vi "main_ctrl.vi"(8 "error in":errorcluster) -> (0 "error out":errorcluster caption="Error")   [LabVIEW 2013]
uses:
  <vilib>/Rock Robotics/WPI/DriverStation/WPI_DriverStationRobotMode2.ctl
  typedefs/fg_typedef.ctl
  typedefs/vision enable.ctl
  typedefs/subStates.ctl
  typedefs/singleUseSubstate.ctl
  <vilib>/Rock Robotics/WPI/Solenoid/WPI_SolenoidValue.ctl
  <vilib>/Rock Robotics/WPI/Compressor/WPI_CompressorGetSetRefNum.vi
  <vilib>/Rock Robotics/WPI/RobotDrive/WPI_RobotDriveGetSetRefNum.vi
  <vilib>/Rock Robotics/WPI/RobotDrive/WPI_RobotDriveArcadeDrive_Standard(NoSaturation).vi
  <vilib>/Rock Robotics/WPI/Solenoid/WPI_SolenoidSetEnum.vi
  typedefs/vision data.ctl
panel:
  out "Robot Mode":T1
  out "Vision SPI":u32
  out "Vision IPS":dbl
  out "Main IPS":dbl
  out "Main SPI":u32
  # "MAIN CONTROL"
  # "holds robot control code - dual parallel state machine"
  # "SPI: milliseconds per iteration\nIPS: iterations per second"
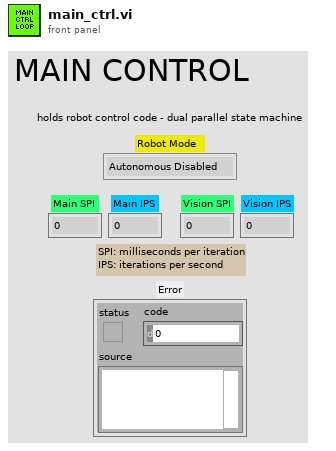
[diagram p1: front panel]
types:
  T1 = typedef "WPI_DriverStationRobotMode2.ctl" = enum16{"Autonomous Disabled", "Autonomous Enabled", "Teleop Disabled", "Teleop Enabled", "Timeout", "Finish", "Test Disabled", "Test Enabled"}
  T2 = typedef "fg_typedef.ctl" = enum16{"Get", "Set"}
  T3 = typedef "WPI_DigitalInputDevRef.ctl" = cluster{"DevStatus":errorcluster, "DIO Channel":T4, "Digital Module":T5}
  T4 = typedef "FPGA_DIOChannel.ctl" = enum8{"DIO 1", "DIO 2", "DIO 3", "DIO 4", "DIO 5", "DIO 6", "DIO 7", "DIO 8", "DIO 9", "DIO 10", "DIO 11", "DIO 12", "DIO 13", "DIO 14", "Invalid"}
  T5 = typedef "FPGA_TypedefDigitalModule.ctl" = enum16{"Digital Module 1", "Digital Module 2"}
  T6 = typedef "WPI_RobotDriveDevRef.ctl" = cluster{"DevStatus":errorcluster, "Motors[]":T7[], "Square Inputs":bool, "Max Output":dbl, "Isochronous":bool}
  T7 = typedef "WPI_MotorControlDeviceRef.ctl" = cluster{"DeviceStatus":errorcluster, "Type":enum16{"PWM", "CAN"}, "PWM":cluster{"Digital Module":T5, "PWM Channel":T8, "DeadBand":T9}, "CAN":cluster{"Device Number":u8, "Control Mode":T10, "Semaphore":T11, "Max Vout":dbl}, "Invert":bool, "TransformRef":T12, "InvTransformRef":T12}
  T8 = typedef "FPGA_DIOPWMChannel.ctl" = enum8{"PWM 1", "PWM 2", "PWM 3", "PWM 4", "PWM 5", "PWM 6", "PWM 7", "PWM 8", "PWM 9", "PWM 10", "Invalid"}
  T9 = typedef "WPI_PWMDeadband.ctl" = cluster{"Name":string, "maxPositivePwm":i32, "minPositivePwm":i32, "centerPwm":i32, "maxNegativePwm":i32, "minNegativePwm":i32, "angularRange":u16}
  T10 = typedef "WPI_CANJaguar_ControlMode.ctl" = enum8{"Percent VBus", "Current", "Speed", "Position", "Voltage"}
  T11 = typedef "Semaphore RefNum" = refnum<k1>
  T12 = typedef "WPI_PWMTransform_ConPane.ctl" = refnum<vi>
  T13 = typedef "WPI_SolenoidDevRef.ctl" = cluster{"DevStatus":errorcluster, "Solenoid Module":T14, "Forward Solenoid Channel":T15, "Reverse Solenoid Channel":T15}
  T14 = typedef "FPGA_TypedefSolenoidModule.ctl" = enum16{"Solenoid Module 1", "Solenoid Module 2"}
  T15 = typedef "WPI_SolenoidChannel.ctl" = enum8{"Solenoid 1", "Solenoid 2", "Solenoid 3", "Solenoid 4", "Solenoid 5", "Solenoid 6", "Solenoid 7", "Solenoid 8", "Invalid"}
  T16 = typedef "WPI_EncoderDevRef.ctl" = cluster{"DevStatus":errorcluster, "EncoderIndex":T17, "CounterIndex":T18, "DistancePerCount":dbl, "Decoding Type":T19}
  T17 = typedef "FPGA_EncoderIdx.ctl" = enum8{"Enc 0", "Enc 1", "Enc 2", "Enc 3", "Invalid"}
  T18 = typedef "FPGA_CounterCtrSystemIndex.ctl" = enum8{"Ctr 0", "Ctr 1", "Ctr 2", "Ctr 3", "Ctr 4", "Ctr 5", "Ctr 6", "Ctr 7", "Invalid"}
  T19 = typedef "WPI_EncoderType.ctl" = enum16{"1x", "2x", "4x"}
  T20 = typedef "vision data.ctl" = cluster{"x":dbl, "y":dbl, "area":dbl, "width":dbl, "height":dbl, "Hot Goal Present?":bool, "distance":dbl}
  T21 = typedef "vision enable.ctl" = enum16{"Enable", "Disable", "Stop"}
  T22 = typedef "WPI_CameraDevRef.ctl" = cluster{"Camera Address":string, "CameraStatus":errorcluster, "Acquire Image Notifier":refnum<notifier>}
  T23 = typedef "IMAQ Image.ctl" = refnum<image>
  T24 = cluster{"Vision mSPI":u32, "Main mSPI":u32, "Dash mSPI":u32}
  T25 = typedef "WPI_CompressorDevRef.ctl" = cluster{"DevStatus":errorcluster, "DigitalInputDevRef":T3, "RelayDevRef":T26}
  T26 = typedef "WPI_RelayDevRef.ctl" = cluster{"DevStatus":errorcluster, "Relay Channel":T27, "Digital Module":T5, "Relay Direction":T28}
  T27 = typedef "FPGA_DIORelayChannel.ctl" = enum8{"Relay 1", "Relay 2", "Relay 3", "Relay 4", "Relay 5", "Relay 6", "Relay 7", "Relay 8", "Invalid"}
  T28 = typedef "WPI_RelayDirection.ctl" = enum16{"Both directions", "Forward only", "Reverse only"}
  T29 = typedef "WPI_SolenoidValue.ctl" = enum16{"Off", "On", "Forward", "Reverse"}
  T30 = typedef "singleUseSubstate.ctl" = enum16{"null", "wait", "shift high", "shift low", "extend shooter", "retract shooter", "latch", "unlatch", "end"}
  T31 = typedef "WPI_DriverStationDerivedRobotMode.ctl" = enum16{"Init", "Execute", "Stop"}
  T32 = typedef "subStates.ctl" = enum16{"null", "wait", "driver control", "auto", "manual override", "hold position", "rotate", "pickup", "pass", "load", "goto shoot", "shoot high goal", "shoot low goal", "cancel arm", "cancel shooter", "end"}
  T33 = typedef "Loop 2 Datatype.ctl" = cluster{"State":T32, "Waiting Loop":i32, "State to Wait For":i32, "Loop ID":i32, "Exit Value":i32, "Joystick Y":dbl, "Joystick Z":dbl}
  T34 = typedef "Loop 1 Datatype.ctl" = cluster{"State":T32, "Waiting Loop":i32, "State to Wait For":i32, "Loop ID":i32, "Exit Value":i32}
  T35 = typedef "Loop 3 Datatype.ctl" = cluster{"State":T32, "Waiting Loop":i32, "State to Wait For":i32, "Loop ID":i32, "Exit Value":i32, "Joystick Y":dbl, "Tune Setpoint":cluster{"Increment":bool, "Decrement":bool}}
  T36 = typedef "Loop 0 Datatype.ctl" = cluster{"State":T32, "Waiting Loop":i32, "State to Wait For":i32, "Loop ID":i32, "Exit Value":i32, "X Axis":dbl, "Y Axis":dbl, "Z Axis":dbl}
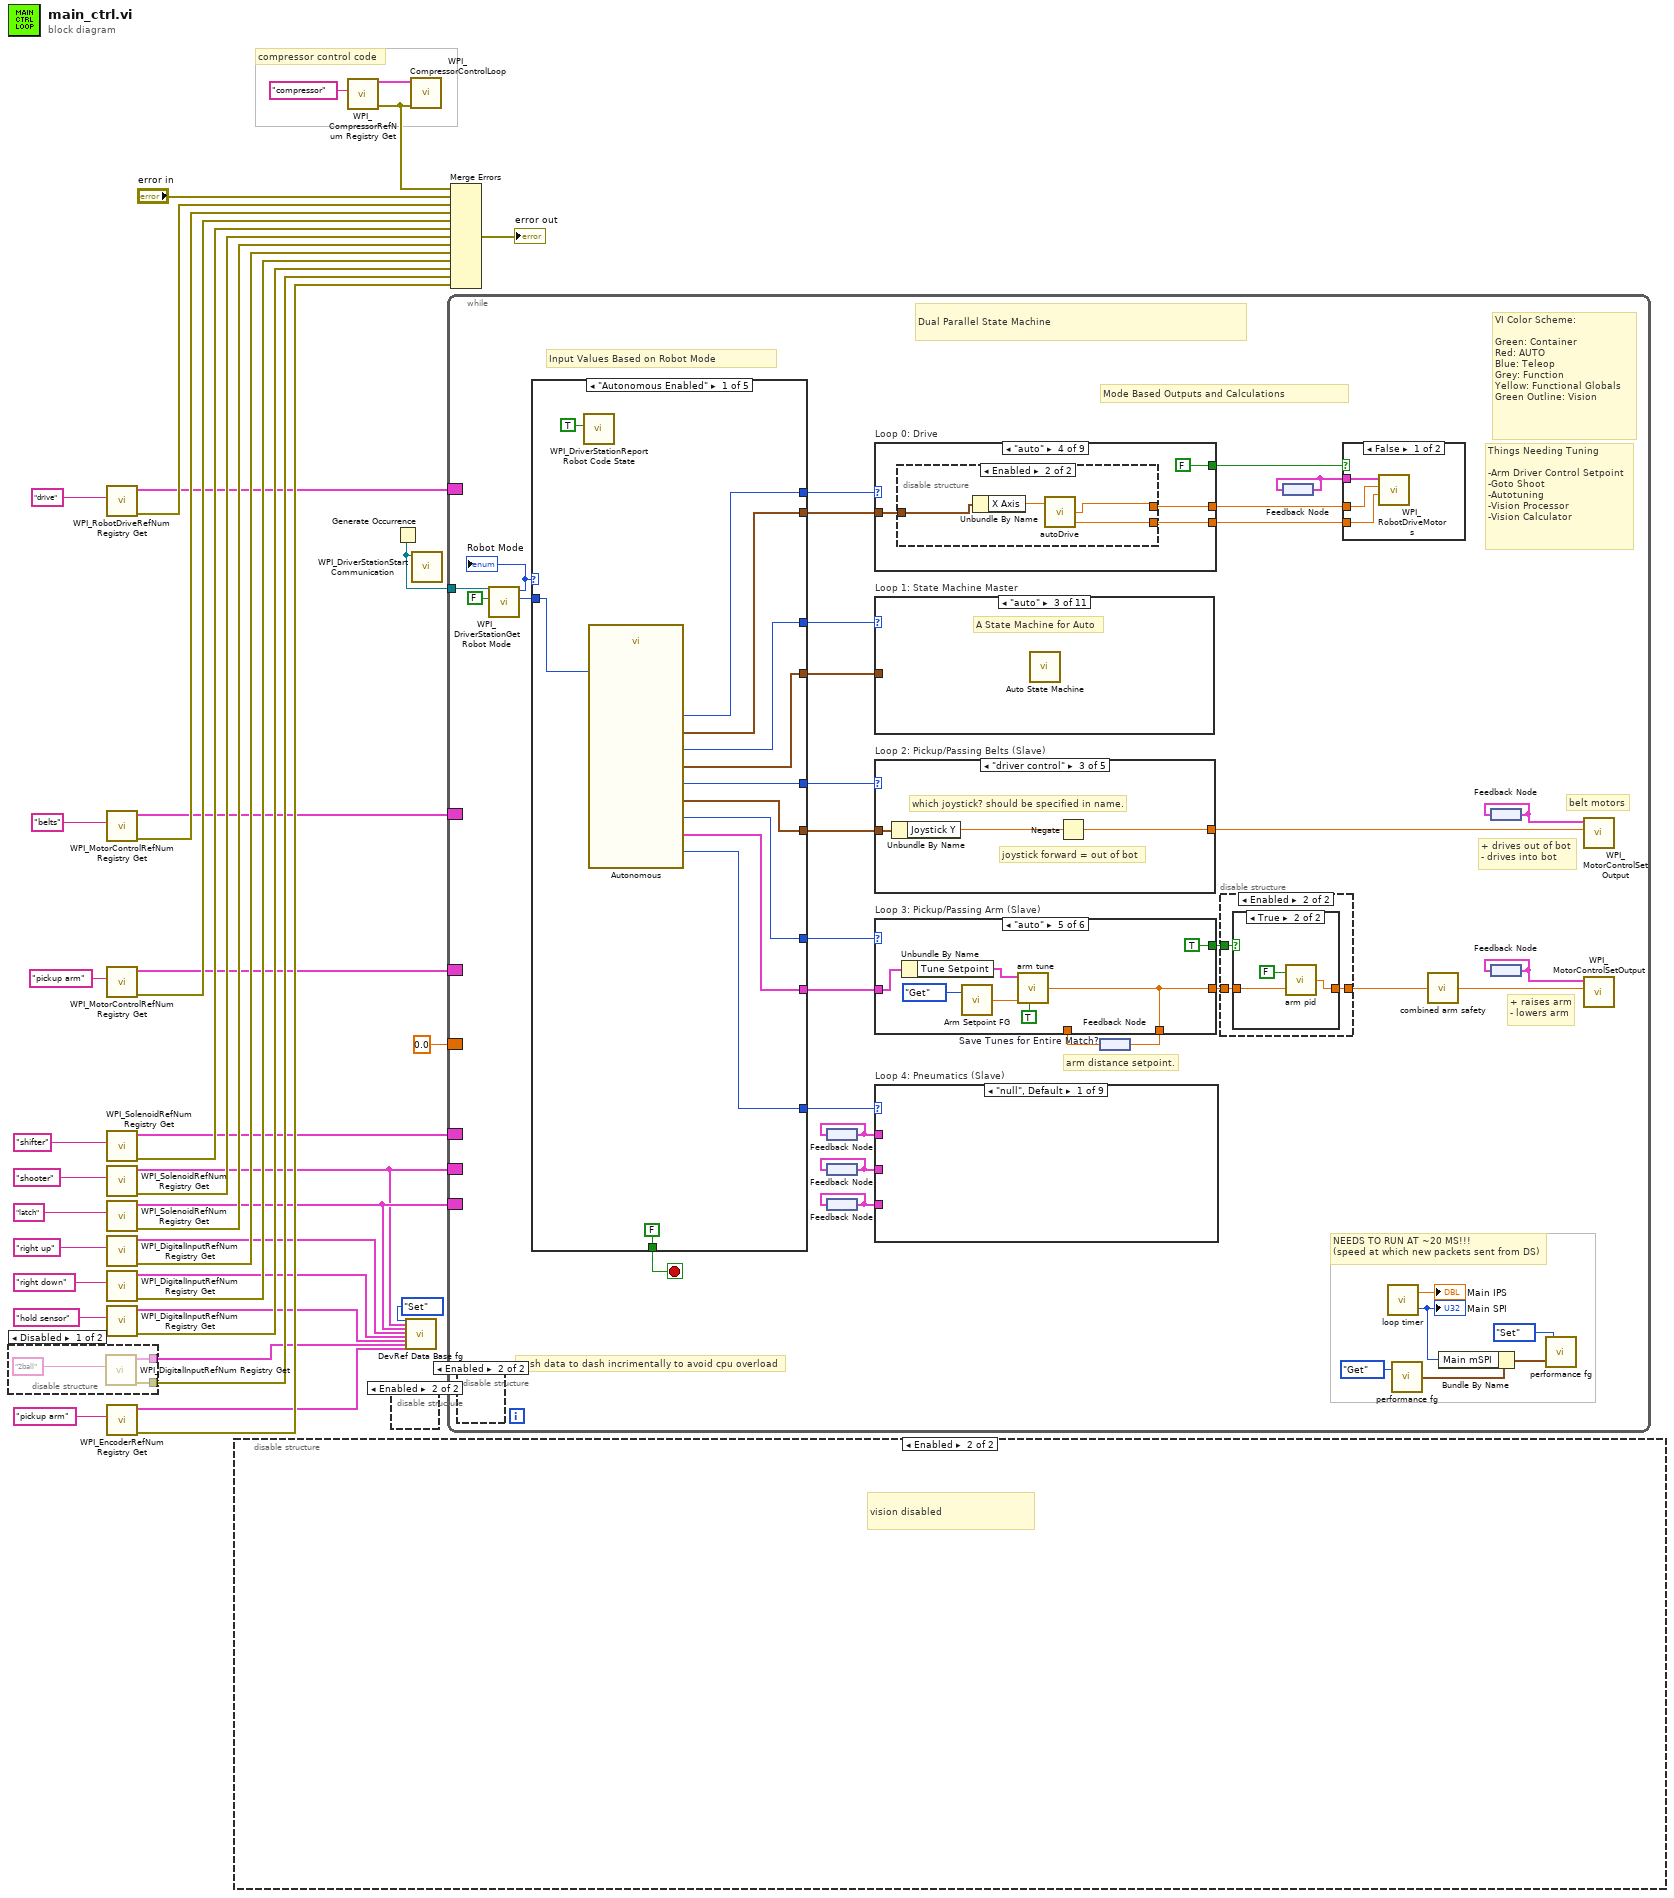
[diagram p0: block diagram]
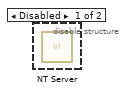
[diagram p3: hidden frame]
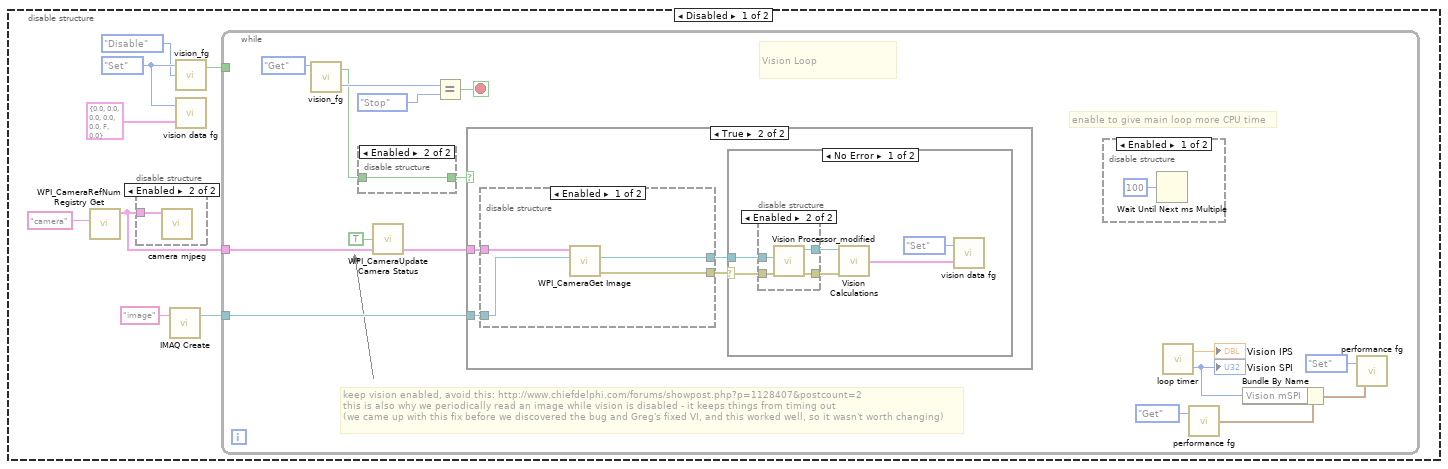
[diagram p4: hidden frame]
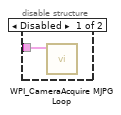
[diagram p5: hidden frame]
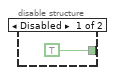
[diagram p6: hidden frame]
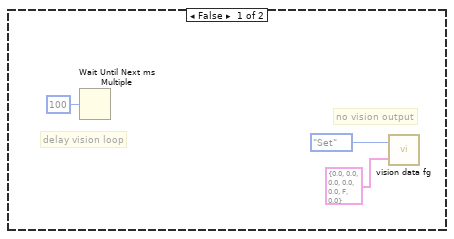
[diagram p8: hidden frame]
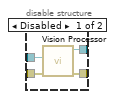
[diagram p9: hidden frame]
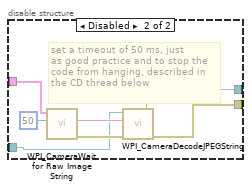
[diagram p11: hidden frame]
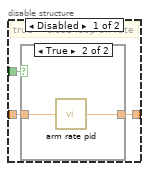
[diagram p12: hidden frame]
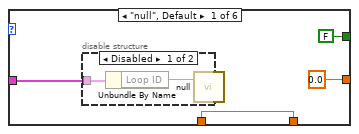
[diagram p15: hidden frame]
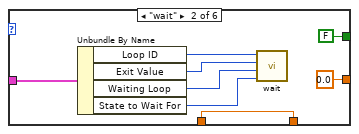
[diagram p17: hidden frame]
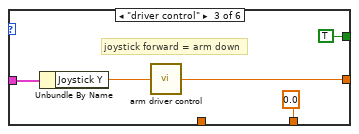
[diagram p18: hidden frame]
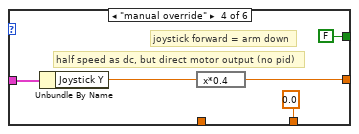
[diagram p19: hidden frame]
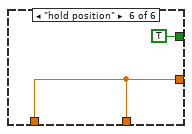
[diagram p20: hidden frame]
diagram:
  # "compressor control code"
  n1 = disable-structure shown="Disabled" {
    disable-tunnel: [w43 _] -> w39
    disable-tunnel: [w41 _] -> w7
    frame Disabled {
      n2 = call <vilib>:"WPI_DigitalInputRefNum Registry Get.vi"("refnum name"="2ball") -> ("error out"=w43:errorcluster, "DigitalInputDevRef"=w41:T3)  [unwired: 9 in]
    }
    frame Enabled {
    }
  }
  n3 = call <vilib>:"WPI_RobotDriveRefNum Registry Get.vi"("refnum name"="drive") -> ("error out"=w38:errorcluster, "RobotDriveDevRef"=w26:T6)  [unwired: 9 in]
  n4 = call <vilib>:"WPI_MotorControlRefNum Registry Get.vi"("refnum name"="belts") -> ("error out"=w37:errorcluster, "MotorControlDevRef"=w5:T7)  [unwired: 9 in]
  n5 = call <vilib>:"WPI_MotorControlRefNum Registry Get.vi"("refnum name"="pickup arm") -> ("error out"=w36:errorcluster, "MotorControlDevRef"=w17:T7)  [unwired: 9 in]
  n6 = call <vilib>:"WPI_SolenoidRefNum Registry Get.vi"("refnum name"="shifter") -> ("error out"=w35:errorcluster, "SolenoidDevRef"=w24:T13)  [unwired: 9 in]
  n7 = call <vilib>:"WPI_SolenoidRefNum Registry Get.vi"("refnum name"="shooter") -> ("error out"=w34:errorcluster, "SolenoidDevRef"=w3:T13)  [unwired: 9 in]
  n8 = call <vilib>:"WPI_SolenoidRefNum Registry Get.vi"("refnum name"="latch") -> ("error out"=w33:errorcluster, "SolenoidDevRef"=w4:T13)  [unwired: 9 in]
  n9 = call <vilib>:"WPI_DigitalInputRefNum Registry Get.vi"("refnum name"="right up") -> ("error out"=w32:errorcluster, "DigitalInputDevRef"=w2:T3)  [unwired: 9 in]
  n10 = call <vilib>:"WPI_DigitalInputRefNum Registry Get.vi"("refnum name"="right down") -> ("error out"=w31:errorcluster, "DigitalInputDevRef"=w1:T3)  [unwired: 9 in]
  n11 = call <vilib>:"WPI_DigitalInputRefNum Registry Get.vi"("refnum name"="hold sensor") -> ("error out"=w30:errorcluster, "DigitalInputDevRef"=w11:T3)  [unwired: 9 in]
  n12 = call <vilib>:"WPI_EncoderRefNum Registry Get.vi"("refnum name"="pickup arm") -> ("error out"=w40:errorcluster, "EncoderDevRef"=w6:T16)  [unwired: 9 in]
  n13 = disable-structure shown="Enabled" {
    frame Disabled {
      w49 = fg_typedef."Set" ("Enum")
      n14 = call <vilib>:"WPI_CameraRefNum Registry Get.vi"("refnum name"="camera") -> ("CameraDevRef"=w46:T22)  [unwired: 9 in, 1 out]
      n15 = disable-structure shown="Enabled" {
        disable-tunnel: w46 -> [w52 w53]
        frame Disabled {
          n16 = call <vilib>:"WPI_CameraAcquire MJPG Loop.vi"("CameraDevRef"=w52) -> ()  [unwired: 11 in]
        }
        frame Enabled {
          n17 = call "camera mjpeg.vi"("CameraDevRef"=w53) -> ()  [unwired: 11 in]
        }
      }
      n18 = call "IMAQ Create"("Image Name"="image") -> ("New Image"=w51:T23)  [unwired: 4 in, 1 out]
      n19 = call "vision_fg.vi"("Action"=vision_enable."Disable", "Menu"=w49) -> ("Enabled?"=w50:bool)  [unwired: 1 in, 1 out]
      n20 = call "vision data fg.vi"("Input"=T20 {"x"=0.0, "y"=0.0, "area"=0.0, "width"=0.0, "height"=0.0, "Hot Goal Present?"=FALSE, "distance"=0.0} ("Cluster"), "Menu"=w49) -> ()  [unwired: 1 out]
      n21 = while {
        tunnel: w51 -> [w68]
        tunnel: w46 -> [w67]
        tunnel: w50 -> [_]
        stop <- w69 stop-if-true
        # "keep vision enabled, avoid this: http://www.chiefdelphi.com/forums/showpost.php?p=1128407&postcount=2\nthis is also why we periodically read an image while vision is disabled - it keeps things from timing out\n(we came up with this fix before we discovered the bug and Greg's fixed VI, and this worked well, so it wasn't worth changing)"
        # "enable to give main loop more CPU time"
        # "Vision Loop"
        n22 = call "vision_fg.vi"("Menu"=fg_typedef."Get" ("Enum")) -> ("State Out"=w63:T21, "Enabled?"=w54:bool)  [unwired: 2 in]
        n23 = disable-structure shown="Enabled" {
          disable-tunnel: [TRUE w71] -> w55
          disable-tunnel: w54 -> [_ w71]
          frame Disabled {
          }
          frame Enabled {
          }
        }
        n24 = call <vilib>:"WPI_CameraUpdate Camera Status.vi"("CameraDevRef In"=w67, "Enable Vision"=TRUE) -> ("CameraDevRef Out"=w66:T22)  [unwired: 3 in]
        n25 = Equal?(x=w63, y=vision_enable."Stop") -> (x = y?=w69:bool)
        n26 = case shown="True" w55 {
          tunnel: w68 -> [_ w79]
          tunnel: w66 -> [_ w78]
          frame False {
            # "no vision output"
            # "delay vision loop"
            n27 = Wait Until Next ms Multiple(millisecond multiple=u32 100) -> ()  [unwired: 1 out]
            n28 = call "vision data fg.vi"("Input"=T20 {"x"=0.0, "y"=0.0, "area"=0.0, "width"=0.0, "height"=0.0, "Hot Goal Present?"=FALSE, "distance"=0.0} ("Cluster"), "Menu"=fg_typedef."Set" ("Enum")) -> ()  [unwired: 1 out]
          }
          frame True {
            n29 = disable-structure shown="Enabled" {
              disable-tunnel: w79 -> [w96 w100]
              disable-tunnel: w78 -> [w97 w102]
              disable-tunnel: [w95 w99] -> w77
              disable-tunnel: [w94 w98] -> w76
              frame Enabled {
                n30 = call <vilib>:"WPI_CameraGet Image.vi"("Image"=w96, "CameraDevRef"=w97) -> ("error out"=w94:errorcluster, "Image Out"=w95:T23)  [unwired: 7 in, 1 out]
              }
              frame Disabled {
                # "set a timeout of 50 ms, just\nas good practice and to stop the \ncode from hanging, described in \nthe CD thread below"
                n31 = call <vilib>:"WPI_CameraWait for Raw Image String.vi"("Timeout in ms (-1)"=50, "CameraDevRef"=w102) -> ("error out"=w104:errorcluster, "String"=w103:string)  [unwired: 3 in, 5 out]
                n32 = call <vilib>:"WPI_CameraDecodeJPEGString.vi"("error in"=w104, "Compressed Image"=w103, "Image In"=w100) -> ("error out"=w98:errorcluster, "Image Out"=w99:T23)  [unwired: 3 out]
              }
            }
            n33 = case shown="No Error" w76 {
              selector: w76 -> [w84 _]
              tunnel: w77 -> [w83 _]
              frame No Error {
                n34 = disable-structure shown="Enabled" {
                  disable-tunnel: w84 -> [w89 w92]
                  disable-tunnel: w83 -> [w88 w93]
                  disable-tunnel: [w87 w90] -> w82
                  disable-tunnel: [w86 w91] -> w81
                  frame Disabled {
                    n35 = call "Vision Processor.vi"("error in"=w89, "Image In"=w88) -> ("error out"=w86:errorcluster, "Image Out"=w87:T23)  [unwired: 5 in]
                  }
                  frame Enabled {
                    n36 = call "Vision Processor_modified.vi"("error in"=w92, "Image In"=w93) -> ("error out"=w91:errorcluster, "Image Out"=w90:T23)  [unwired: 5 in]
                  }
                }
                n37 = call "Vision Calculations.vi"("Image In"=w82, "error in"=w81) -> ("Vision Data"=w80:T20)  [unwired: 3 in]
                n38 = call "vision data fg.vi"("Input"=w80, "Menu"=fg_typedef."Set" ("Enum")) -> ()  [unwired: 1 out]
              }
              frame Error {
              }
            }
          }
        }
        n39 = disable-structure shown="Enabled" {
          frame Enabled {
            n40 = Wait Until Next ms Multiple(millisecond multiple=u32 100) -> ()  [unwired: 1 out]
          }
          frame Disabled {
          }
        }
        n41 = call "loop timer.vi"() -> ("IPS"=→"Vision IPS":dbl, "SPI"=w61:u32)  [unwired: 1 in]
        "Vision SPI" <- w61
        n42 = call "performance fg.vi"("Menu"=fg_typedef."Get") -> ("Output"=w59:T24)  [unwired: 1 in]
        n43 = Bundle By Name(cluster=w59, "Vision mSPI"=w61) -> (w58:T24)
        n44 = call "performance fg.vi"("Input"=w58, "Menu"=fg_typedef."Set") -> ()  [unwired: 1 out]
      }
    }
    frame Enabled {
      # "vision disabled"
    }
  }
  n45 = call <vilib>:"WPI_CompressorRefNum Registry Get.vi"("refnum name"="compressor") -> ("error out"=w10:errorcluster, "CompressorDevRef"=w25:T25)  [unwired: 9 in]
  n46 = disable-structure shown="Enabled" {
    frame Disabled {
      n47 = call <vilib>:"NT Server.vi"() -> ()  [unwired: 12 in]
    }
    frame Enabled {
    }
  }
  n48 = Generate Occurrence() -> (w22:refnum<k4>)
  n49 = call "DevRef Data Base fg.vi"("Menu"=fg_typedef."Set", "Shooter Solenoid DevRef"=w3, "Latch Solenoid DevRef"=w4, "Right Up DevRef"=w2, "Right Down DevRef"=w1, "Hold Sensor DevRef"=w11, "2 Ball DevRef"=w7, "Arm Encoder DevRef"=w6) -> ()  [unwired: 17 in, 3 out]
  n50 = call <vilib>:"WPI_CompressorControlLoop.vi"("error in (no error)"=w10, "CompressorDevRef"=w25) -> ()  [unwired: 10 in]
  n51 = call <vilib>:"WPI_DriverStationStart Communication.vi"("occurrence"=w22) -> ()  [unwired: 11 in]
  n52 = while {
    tunnel: w22 -> [w120]
    border: w26 -> [_]
    border: w24 -> [_]
    border: w4 -> [_]
    border: w3 -> [_]
    border: w5 -> [_]
    border: w17 -> [_]
    border: 0.0 ("setpoint") -> [_]
    stop <- w137 stop-if-true
    # "arm distance setpoint."
    # "push data to dash incrimentally to avoid cpu overload"
    # "Things Needing Tuning\n\n-Arm Driver Control Setpoint\n-Goto Shoot\n-Autotuning\n-Vision Processor\n-Vision Calculator"
    # "+ raises arm\n- lowers arm"
    # "+ drives out of bot\n- drives into bot"
    # "belt motors"
    # "VI Color Scheme:\n\nGreen: Container\nRed: AUTO\nBlue: Teleop\nGrey: Function\nYellow: Functional Globals\nGreen Outline: Vision"
    # "Input Values Based on Robot Mode"
    # "Mode Based Outputs and Calculations"
    # "NEEDS TO RUN AT ~20 MS!!!\n(speed at which new packets sent from DS)"
    # "Dual Parallel State Machine"
    n53 = disable-structure shown="Enabled" {
      frame Disabled {
        n54 = call "BuildCustomDashBoardData.vi"() -> ()  [unwired: 12 in]
      }
      frame Enabled {
      }
    }
    n55 = call <vilib>:"WPI_DriverStationGet Robot Mode.vi"("Finish"=FALSE, "DS Occurrence"=w120) -> ("Call Context"=w119:T31, "Robot Mode"=w118:T1)  [unwired: 8 out]
    "Robot Mode" <- w118
    n56 = case shown="\"Autonomous Enabled\"" w118 {
      tunnel: [w324 w339 w342 w348 w354] -> w122
      tunnel: w119 -> [w317 w335 _ _ _]
      tunnel: [w322 w338 w342 w348 w354] -> w139
      tunnel: [w318 w336 singleUseSubstate."null" ("SubState 5") singleUseSubstate."null" ("SubState 5") singleUseSubstate."end" ("SubState 5")] -> w138
      tunnel: [FALSE FALSE FALSE FALSE TRUE] -> w137
      tunnel: [w326 w334 w342 w348 w354] -> w106
      tunnel: [w325 w333 _ _ _] -> w131
      tunnel: [w323 w332 _ _ _] -> w130
      tunnel: [w321 w331 _ _ _] -> w129
      tunnel: [w319 w330 _ _ _] -> w127
      tunnel: [w320 w329 w342 w348 w354] -> w105
      frame "Autonomous Enabled" {
        n57 = call <vilib>:"WPI_DriverStationReport Robot Code State.vi"("Autonomous"=TRUE) -> ()  [unwired: 10 in, 1 out]
        n58 = call "Autonomous.vi"("Call Context"=w317) -> ("SubState 2"=w322:T32, "Loop 2 Data"=w321:T33, "SubState 1"=w324:T32, "Loop 1 Data"=w323:T34, "Loop 3 Data"=w319:T35, "SubState 0"=w326:T32, "SubState 3"=w320:T32, "Loop 0 Data"=w325:T36, "SubState 4"=w318:T30)  [unwired: 2 in]
      }
      frame "Teleop Enabled" {
        n59 = call <vilib>:"WPI_DriverStationReport Robot Code State.vi"("TeleOp"=TRUE) -> ()  [unwired: 10 in, 1 out]
        n60 = call "Teleop.vi"("Call Context"=w335) -> ("SubState 3"=w329:T32, "SubState 4"=w336:T30, "Loop 3 Data"=w330:T35, "SubState 0"=w334:T32, "Loop 1 Data"=w332:T34, "Loop 0 Data"=w333:T36, "SubState 1"=w339:T32, "Loop 2 Data"=w331:T33, "SubState 2"=w338:T32)  [unwired: 10 in]
      }
      frame "Autonomous Disabled", "Teleop Disabled", "Timeout" {
        w342 = subStates."null" ("SubState 0")
        # "set all loops to null"
        # "make sure to disable vision\nwe don't need it here"
        # "robot disabled, timeout"
        n61 = call <vilib>:"WPI_DriverStationReport Robot Code State.vi"("Disabled"=TRUE) -> ()  [unwired: 10 in, 1 out]
        n62 = call "vision_fg.vi"("Action"=vision_enable."Disable", "Menu"=fg_typedef."Set") -> ()  [unwired: 1 in, 2 out]
      }
      frame "Test Disabled", "Test Enabled" {
        w348 = subStates."null" ("SubState 0")
        # "set all loops to null"
        # "make sure to disable vision\nwe don't need it here"
        # "test, unused"
        n63 = call <vilib>:"WPI_DriverStationReport Robot Code State.vi"("Test"=TRUE) -> ()  [unwired: 10 in, 1 out]
        n64 = call "vision_fg.vi"("Action"=vision_enable."Disable", "Menu"=fg_typedef."Set") -> ()  [unwired: 1 in, 2 out]
      }
      frame "Finish" {
        w354 = subStates."end"  # Stop All Loops
        # "stop the while loop"
        # "stop DS comms"
        # "stop vision loop"
        n65 = call <vilib>:"WPI_DriverStationStop Communication.vi"("StopCommunication"=TRUE) -> ()  [unwired: 10 in, 1 out]
        n66 = call "vision_fg.vi"("Action"=vision_enable."Stop", "Menu"=fg_typedef."Set") -> ()  [unwired: 1 in, 2 out]
      }
    }
    n67 = feedback #1() -> (w128:T13)
    n68 = feedback-in #1(w128) -> ()
    n69 = feedback #2() -> (w112:T13)
    n70 = feedback-in #2(w112) -> ()
    n71 = feedback #3() -> (w111:T13)
    n72 = feedback-in #3(w111) -> ()
    n73 = case "Loop 0: Drive" shown="\"auto\"" w106 {
      tunnel: w131 -> [w195 w200 w210 w217 w238 w245 _ _ w263]
      tunnel: [w193 w198 w208 w219 w235 w247 w250 w257 w259] -> w125
      tunnel: [w193 w198 w207 w218 w234 w246 w249 w257 w258] -> w124
      tunnel: [FALSE FALSE TRUE FALSE FALSE FALSE FALSE FALSE FALSE] -> w126
      frame "null", Default {
        w193 = 0.0 ("X Axis")
        n74 = disable-structure shown="Disabled" {
          disable-tunnel: w195 -> [w196 _]
          frame Disabled {
            n75 = Unbundle By Name(w196) -> ("Loop ID"=w197:i32)
            n76 = call "null.vi"("This Loop ID"=w197) -> ()  [unwired: 2 in]
          }
          frame Enabled {
          }
        }
      }
      frame "wait" {
        w198 = 0.0 ("X Axis")
        n77 = Unbundle By Name(w200) -> ("Loop ID"=w204:i32, "Exit Value"=w203:i32, "Waiting Loop"=w202:i32, "State to Wait For"=w201:i32)
        n78 = call "wait.vi"("State to wait for"=w201, "Waiting Loop ID"=w202, "time (ms)"=w203, "Current Loop ID"=w204) -> ()  [unwired: 1 out]
      }
      frame "driver control" {
        n79 = Unbundle By Name(w210) -> ("X Axis"=w205:dbl, "Y Axis"=w206:dbl)
        n80 = disable-structure shown="Enabled" {
          disable-tunnel: w205 -> [w214 w216]
          disable-tunnel: w206 -> [w213 w215]
          disable-tunnel: [w212 w216] -> w208
          disable-tunnel: [w211 w215] -> w207
          frame Disabled {
            n81 = call "calc arcade drive pwm.vi"("Y axis value"=w213, "X axis value"=w214) -> ("Right Speed"=w211:dbl, "Left Speed"=w212:dbl)  [unwired: 1 in, 1 out]
          }
          frame Enabled {
          }
        }
      }
      frame "auto" {
        n82 = disable-structure shown="Enabled" {
          disable-tunnel: [w228 w231] -> w219
          disable-tunnel: [w227 w230] -> w218
          disable-tunnel: w217 -> [w223 w232]
          frame Disabled {
            n83 = Unbundle By Name(w223) -> ("Z Axis"=w221:dbl)
            n84 = call "Vision Tracking X.vi"("Tweak"=w221) -> ("right speed"=w222:dbl, "left speed"=w225:dbl)
            n85 = call "closed drive.vi"("Acrade Drive?"=FALSE, "Y axis value (Left)"=w225, "X axis value (Right)"=w222, "Threshold (.4)"=0.0 ("Threshold")) -> ("right"=w227:dbl, "left"=w228:dbl)
          }
          frame Enabled {
            n86 = Unbundle By Name(w232) -> ("X Axis"=w229:dbl)
            n87 = call "autoDrive.vi"("Distance to Travel"=w229) -> ("left speed"=w231:dbl, "right speed"=w230:dbl)  [unwired: 1 in, 1 out]
          }
        }
      }
      frame "hold position" {
        n88 = Unbundle By Name(w238) -> ("X Axis"=w237:dbl, "Y Axis"=w236:dbl)
        n89 = call "closed drive.vi"("Acrade Drive?"=TRUE, "Y axis value (Left)"=w236, "X axis value (Right)"=w237) -> ("right"=w234:dbl, "left"=w235:dbl)  [unwired: 1 in]
      }
      frame "rotate" {
        # "use these to carry actual information because this is\nfor autonomous only so there will not be joystick input"
        n90 = Unbundle By Name(w245) -> ("X Axis"=w244:dbl, "Y Axis"=w243:dbl)
        n91 = call "rotate.vi"("Angle"=w244, "Rate"=w243) -> ("finished?"=w240:bool, "left speed"=w247:dbl, "right speed"=w246:dbl)
        n92 = call "states FG.vi"("exit in"=w240, "menu (get)"=enum16{"set", "get"}."set", "Loop ID"=0) -> ()  [unwired: 5 in, 4 out]
      }
      frame "goto shoot" {
        n93 = disable-structure shown="Disabled" {
          disable-tunnel: [w253 _] -> w250
          disable-tunnel: [w252 _] -> w249
          frame Disabled {
            # "consider implimenting closed hold with drive"
            n94 = call "vision data fg.vi"("Menu"=fg_typedef."Get") -> ("Output"=w254:T20)  [unwired: 1 in]
            n95 = call "goto location.vi"("Image Data"=w254) -> ("left speed"=w253:dbl, "right speed"=w252:dbl)
          }
          frame Enabled {
            # "not going to do this"
          }
        }
      }
      frame "end" {
        w257 = 0.0 ("X Axis")
      }
      frame "manual override" {
        n96 = Unbundle By Name(w263) -> ("X Axis"=w262:dbl, "Y Axis"=w261:dbl)
        n97 = expression code="x/2"(w262) -> (w259:dbl)
        n98 = expression code="x/2"(w261) -> (w258:dbl)
      }
    }
    n99 = case "Loop 1: State Machine Master" shown="\"auto\"" w122 {
      tunnel: w130 -> [w303 w306 _ _ _ _ _ _ _ _ _]
      frame "null", Default {
        n100 = disable-structure shown="Disabled" {
          disable-tunnel: w303 -> [w304 _]
          frame Disabled {
            n101 = Unbundle By Name(w304) -> ("Loop ID"=w305:i32)
            n102 = call "null.vi"("This Loop ID"=w305) -> ()  [unwired: 2 in]
          }
          frame Enabled {
          }
        }
      }
      frame "wait" {
        n103 = Unbundle By Name(w306) -> ("Loop ID"=w310:i32, "Exit Value"=w309:i32, "Waiting Loop"=w308:i32, "State to Wait For"=w307:i32)
        n104 = call "wait.vi"("State to wait for"=w307, "Waiting Loop ID"=w308, "time (ms)"=w309, "Current Loop ID"=w310) -> ()  [unwired: 1 out]
      }
      frame "auto" {
        # "A State Machine for Auto"
        n105 = call "Auto State Machine.vi"() -> ()  [unwired: 12 in]
      }
      frame "manual override" {
        # "manual shoot"
        n106 = call "single use states FG.vi"("exit in"=TRUE, "substate"=singleUseSubstate."unlatch", "menu (get)"=enum16{"set", "get"}."set") -> ()  [unwired: 5 in, 4 out]
      }
      frame "pickup" {
        # "A State Machine for Pickup"
        n107 = call "Pickup State Machine.vi"() -> ()  [unwired: 12 in]
      }
      frame "pass" {
        # "A State Machine for Passing"
        n108 = call "Pass State Machine.vi"() -> ()  [unwired: 12 in]
      }
      frame "load" {
        # "ball can now (after this) be high or low goal shot"
        # "A State Machine for Loading"
        n109 = call "Load State Machine.vi"() -> ()  [unwired: 12 in]
      }
      frame "shoot high goal" {
        # "A State Machine for High Goal Shooting"
        n110 = call "Shoot High Goal State Machine.vi"() -> ()  [unwired: 12 in]
      }
      frame "shoot low goal" {
        # "A State Machine for Low Goal Shooting"
        n111 = call "Shoot Low Goal State Machine.vi"() -> ()  [unwired: 12 in]
      }
      frame "cancel arm" {
        # "A State Machine for Canceling"
        n112 = call "Cancel State Machine.vi"("What to Cancel"=enum16{"Pickup", "Load"}."Pickup") -> ()
      }
      frame "cancel shooter" {
        # "A State Machine for Canceling"
        n113 = call "Cancel State Machine.vi"("What to Cancel"=enum16{"Pickup", "Load"}."Load") -> ()
      }
    }
    n114 = case "Loop 2: Pickup/Passing Belts (Slave)" shown="\"driver control\"" w139 {
      tunnel: w129 -> [w281 w285 w292 w295 w302]
      tunnel: [0.0 ("output") 0.0 ("output") w290 w293 w299] -> w113
      frame "null", Default {
        # "must stay disabled, it caused errors"
        n115 = disable-structure shown="Disabled" {
          disable-tunnel: w281 -> [w283 _]
          frame Disabled {
            n116 = Unbundle By Name(w283) -> ("Loop ID"=w282:i32)
            n117 = call "null.vi"("This Loop ID"=w282) -> ()  [unwired: 2 in]
          }
          frame Enabled {
          }
        }
      }
      frame "wait" {
        n118 = Unbundle By Name(w285) -> ("Loop ID"=w289:i32, "Exit Value"=w288:i32, "Waiting Loop"=w287:i32, "State to Wait For"=w286:i32)
        n119 = call "wait.vi"("State to wait for"=w286, "Waiting Loop ID"=w287, "time (ms)"=w288, "Current Loop ID"=w289) -> ()  [unwired: 1 out]
      }
      frame "driver control" {
        # "which joystick? should be specified in name."
        # "joystick forward = out of bot"
        n120 = Unbundle By Name(w292) -> ("Joystick Y"=w291:dbl)
        n121 = Negate(x=w291) -> (-x=w290:dbl)
      }
      frame "manual override" {
        # "essentially driver control, but 1/2 speed?"
        # "joystick forward = out of bot"
        n122 = Unbundle By Name(w295) -> ("Joystick Y"=w294:dbl)
        n123 = expression code="-x/2"(w294) -> (w293:dbl)
      }
      frame "auto" {
        # "get speed to go as set by master and tune"
        n124 = Unbundle By Name(w302) -> ("Joystick Z"=w300:dbl)
        n125 = call "Joystick tuner.vi"("Joystick Z"=w300, "Loop ID"=2) -> ("Output"=w298:dbl)  [unwired: 7 in]
        n126 = call "Belt Speed FG.vi"("Menu"=fg_typedef."Get") -> ("Speed Out"=w297:dbl)  [unwired: 1 in]
        n127 = Multiply(x=w298, y=w297) -> (x*y=w299:dbl)
      }
    }
    n128 = case "Loop 4: Pneumatics (Slave)" shown="\"null\", Default" w138 {
      tunnel: w128 -> [_ _ w265 w266 _ _ _ _ _]
      tunnel: w112 -> [_ _ _ _ w268 w270 _ _ w278]
      tunnel: w111 -> [_ _ _ _ _ _ w272 w274 w276]
      frame "null", Default {
      }
      frame "wait" {
      }
      frame "shift high" {
        n129 = call-poly <vilib>:"WPI_SolenoidSet.vi"("Value"=WPI_SolenoidValue."Forward", "SolenoidDevRef"=w265) -> ()  [unwired: 8 in, 2 out]
      }
      frame "shift low" {
        n130 = call-poly <vilib>:"WPI_SolenoidSet.vi"("Value"=WPI_SolenoidValue."Reverse", "SolenoidDevRef"=w266) -> ()  [unwired: 8 in, 2 out]
      }
      frame "extend shooter" {
        n131 = call-poly <vilib>:"WPI_SolenoidSet.vi"("Value"=WPI_SolenoidValue."Forward", "SolenoidDevRef"=w268) -> ()  [unwired: 8 in, 2 out]
      }
      frame "retract shooter" {
        n132 = call-poly <vilib>:"WPI_SolenoidSet.vi"("Value"=WPI_SolenoidValue."Reverse", "SolenoidDevRef"=w270) -> ()  [unwired: 8 in, 2 out]
      }
      frame "latch" {
        # "When the latch piston\nis reversed, the latch\nis closed. When the\nlatch piston is\nextended, the latch is\nopen."
        n133 = call-poly <vilib>:"WPI_SolenoidSet.vi"("Value"=WPI_SolenoidValue."Reverse", "SolenoidDevRef"=w272) -> ()  [unwired: 8 in, 2 out]
      }
      frame "unlatch" {
        # "When the latch piston\nis reversed, the latch\nis closed. When the\nlatch piston is\nextended, the latch is\nopen."
        n134 = call-poly <vilib>:"WPI_SolenoidSet.vi"("Value"=WPI_SolenoidValue."Forward", "SolenoidDevRef"=w274) -> ()  [unwired: 8 in, 2 out]
      }
      frame "end" {
        # "retract shooter and unlatch"
        n135 = call-poly <vilib>:"WPI_SolenoidSet.vi"("Value"=WPI_SolenoidValue."Reverse", "SolenoidDevRef"=w278) -> ()  [unwired: 8 in, 2 out]
        n136 = call-poly <vilib>:"WPI_SolenoidSet.vi"("Value"=WPI_SolenoidValue."Forward", "SolenoidDevRef"=w276) -> ()  [unwired: 8 in, 2 out]
      }
    }
    n137 = feedback #4() -> (w107:dbl)
    n138 = case "Loop 3: Pickup/Passing Arm (Slave)" shown="\"auto\"" w105 {
      tunnel: w127 -> [w157 w163 w171 w177 w184 _]
      tunnel: [FALSE FALSE TRUE FALSE TRUE TRUE] -> w110
      tunnel: [0.0 ("output") 0.0 ("output") w170 w175 w178 w185] -> w109
      tunnel: [w154 w160 0.0 ("setpoint") 0.0 ("setpoint") w178 w185] -> w108
      tunnel: w107 -> [w154 w160 _ _ _ w185]
      frame "null", Default {
        n139 = disable-structure shown="Disabled" {
          disable-tunnel: w157 -> [w159 _]
          frame Disabled {
            n140 = Unbundle By Name(w159) -> ("Loop ID"=w158:i32)
            n141 = call "null.vi"("This Loop ID"=w158) -> ()  [unwired: 2 in]
          }
          frame Enabled {
          }
        }
      }
      frame "wait" {
        n142 = Unbundle By Name(w163) -> ("Loop ID"=w167:i32, "Exit Value"=w166:i32, "Waiting Loop"=w165:i32, "State to Wait For"=w164:i32)
        n143 = call "wait.vi"("State to wait for"=w164, "Waiting Loop ID"=w165, "time (ms)"=w166, "Current Loop ID"=w167) -> ()  [unwired: 1 out]
      }
      frame "driver control" {
        # "joystick forward = arm down"
        n144 = Unbundle By Name(w171) -> ("Joystick Y"=w169:dbl)
        n145 = call "arm driver control.vi"("Joystick Y"=w169) -> ("Setpoint"=w170:dbl)
      }
      frame "manual override" {
        # "half speed as dc, but direct motor output (no pid)"
        # "joystick forward = arm down"
        n146 = Unbundle By Name(w177) -> ("Joystick Y"=w176:dbl)
        n147 = expression code="x*0.4"(w176) -> (w175:dbl)
      }
      frame "auto" {
        w179 = TRUE  # Save Tunes for Entire Match?
        n148 = Unbundle By Name(w184) -> ("Tune Setpoint"=w181:cluster{"Increment":bool, "Decrement":bool})
        n149 = call "Arm Setpoint FG.vi"("Menu"=fg_typedef."Get") -> ("Setpoint Out"=w180:dbl)  [unwired: 1 in]
        n150 = call "arm tune.vi"("Tune Data"=w181, "Setpoint"=w180, "Save Tunes for Entire Match?"=w179) -> ("Tuned Setpoint"=w178:dbl)  [unwired: 4 in]
      }
      frame "hold position" {
      }
    }
    n151 = feedback-in #4(w108) -> ()
    n152 = disable-structure shown="Enabled" {
      disable-tunnel: w110 -> [w143 w149]
      disable-tunnel: w109 -> [w142 w148]
      disable-tunnel: [w141 w147] -> w115
      frame Disabled {
        # "true = close loop on rate"
        n153 = case shown="True" w143 {
          tunnel: w142 -> [w144 w146]
          tunnel: [w144 w145] -> w141
          frame False {
            # "open loop"
          }
          frame True {
            n154 = call "arm rate pid.vi"("Rate In"=w146) -> ("Rate Out"=w145:dbl)
          }
        }
      }
      frame Enabled {
        n155 = case shown="True" w149 {
          tunnel: w148 -> [w150 w152]
          tunnel: [w150 w151] -> w147
          frame False {
            # "open loop"
          }
          frame True {
            n156 = call "arm pid.vi"("Setpoint"=w152, "Autotune?"=FALSE) -> ("Output"=w151:dbl)
          }
        }
      }
    }
    n157 = feedback #5() -> (w123:T6)
    n158 = feedback-in #5(w123) -> ()
    n159 = case shown="False" w126 {
      tunnel: w125 -> [w188 w192]
      tunnel: w124 -> [w187 w191]
      tunnel: w123 -> [w189 w190]
      frame False {
        n160 = call <vilib>:"WPI_RobotDriveMotors.vi"("RightSpeed"=w187, "LeftSpeed"=w188, "RobotDriveDevRef"=w189) -> ()  [unwired: 6 in, 3 out]
      }
      frame True {
        n161 = call-poly <vilib>:"WPI_RobotDriveArcadeDrive.vi"("Y axis value"=w191, "X axis value"=w192, "RobotDriveDevRef"=w190) -> ()  [unwired: 6 in, 3 out]
      }
    }
    n162 = call "loop timer.vi"() -> ("IPS"=→"Main IPS":dbl, "SPI"=w136:u32)  [unwired: 1 in]
    "Main SPI" <- w136
    n163 = call "performance fg.vi"("Menu"=fg_typedef."Get") -> ("Output"=w133:T24)  [unwired: 1 in]
    n164 = call "combined arm safety.vi"("Input"=w115) -> ("Safe Output"=w114:dbl)  [unwired: 13 in, 1 out]
    n165 = Bundle By Name(cluster=w133, "Main mSPI"=w136) -> (w132:T24)
    n166 = feedback #6() -> (w117:T7)
    n167 = feedback-in #6(w117) -> ()
    n168 = feedback #7() -> (w116:T7)
    n169 = feedback-in #7(w116) -> ()
    n170 = call "performance fg.vi"("Input"=w132, "Menu"=fg_typedef."Set") -> ()  [unwired: 1 out]
    n171 = call <vilib>:"WPI_MotorControlSetOutput.vi"("Output"=w113, "MotorControlDevRef"=w117) -> ()  [unwired: 7 in, 3 out]
    n172 = call <vilib>:"WPI_MotorControlSetOutput.vi"("Output"=w114, "MotorControlDevRef"=w116) -> ()  [unwired: 7 in, 3 out]
  }
  n173 = Merge Errors(w10, "error in", w38, w37, w36, w35, w34, w33, w32, w31, w30, w39, w40) -> (→"error out":errorcluster)
